vi "new_document.vi"(8 "Path to creds.json file":path=path "/Users/milandahal/Documents/GitHub/Onshape/python/creds.json", 11 "Name":string) -> (0 "Output Body":string, 3 "Output headers":string)   [LabVIEW 2019]
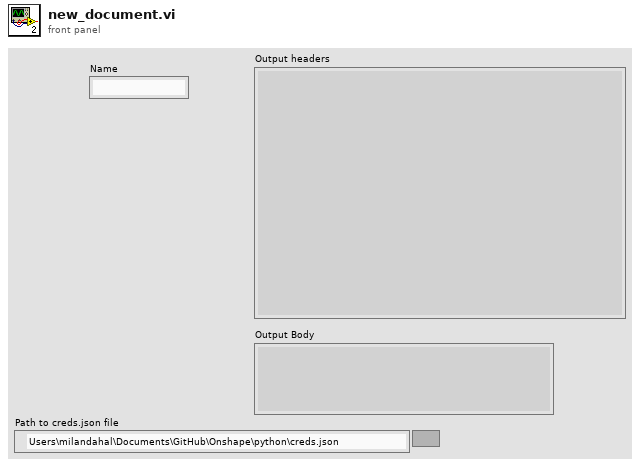
[diagram p1: front panel]
types:
  T1 = cluster{"name":string, "ownerType":i32, "isPublic":bool}
  T2 = cluster{"Date":string, "On-Nonce":string, "ctype":string, "path":string, "method":string, "Authorization":string, "Accept":string, "User-Agent":string, "Content-Type":string, "secret_key":string, "access_key":string, "stack":string, "payload":string}
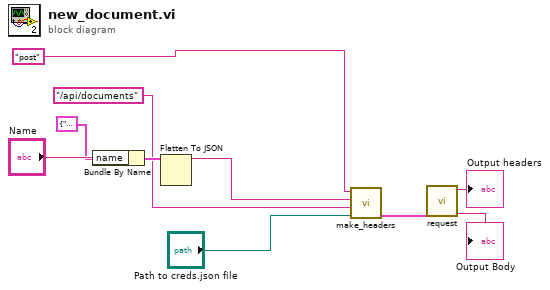
[diagram p0: block diagram]
diagram:
  n1 = Bundle By Name(cluster=T1 {"name"="milan", "ownerType"=0, "isPublic"=FALSE}, "name"="Name") -> (w9:T1)
  n2 = Flatten To JSON(anything=w9) -> (JSON string=w2:string)  [unwired: 2 in, 1 out]
  n3 = call "make_headers.vi"("Method"="post", "payload"=w2, "path"="/api/documents" ("payload"), "Path to creds.json file"="Path to creds.json file") -> ("output cluster"=w7:T2)  [unwired: 5 in, 1 out]
  n4 = call "request.vi"("input cluster"=w7) -> ("Output headers"=→"Output headers":string, "Output Body"=→"Output Body":string)  [unwired: 7 in]
